vi "DisableButton.vi"(8 "error in (no error)":errorcluster, 11 "Boolean in":refnum<vi>) -> (0 "error out":errorcluster)   [LabVIEW 2018]
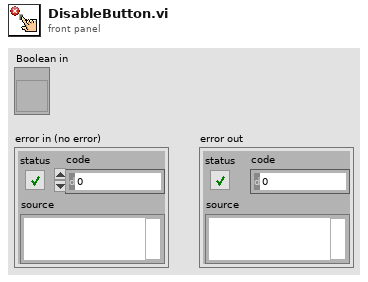
[diagram p1: front panel]
types:
  T1 = enum8{"Enabled", "Disabled", "Disabled and Grayed Out"}
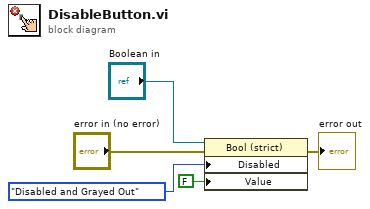
[diagram p0: block diagram]
diagram:
  n1 = property on="Property Node" class="Bool (strict)"(reference="Boolean in", error in="error in (no error)", "Disabled"=T1."Disabled and Grayed Out", "Value"=FALSE) -> (error out=→"error out":errorcluster)  [unwired: 1 out]
